vi "ParameterParser3.vi"() -> ()   [LabVIEW 2019]
panel:
  out "Parmeter Array":string[](array[string])
  in  "Parameter String":string
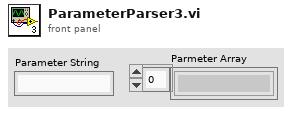
[diagram p1: front panel]
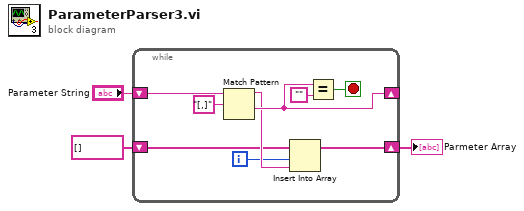
[diagram p0: block diagram]
diagram:
  n1 = while {
    shift-right: [w8] -> _
    shift-left: "Parameter String" -> [w11]
    shift-right: [w7] -> w1
    shift-left: string[] [] -> [w5]
    i -> [w4]
    stop <- w9 stop-if-true
    n2 = Match Pattern(string=w11, regular expression="[,]") -> (before substring=w6:string, after substring=w8:string)  [unwired: 1 in, 2 out]
    n3 = Insert Into Array(array=w5, index=w4, new element=w6) -> (w7:string[])
    n4 = Equal?(x=w8, y="") -> (x = y?=w9:bool)
  }
  "Parmeter Array" <- w1
